vi "DtCreateAoutRawChan.vi"(2 "Range Min":dbl=-10.0, 3 "Range Max":dbl=10.0, 5 "Board Name":string, 7 "Channel":string="0", 9 "Element":u32, 11 "error in (no error)":errorcluster) -> (4 "Task out":i32, 8 "Actual Number of Channels":u32, 15 "error out":errorcluster)   [LabVIEW 2016]
doc: "Creates one or more virtual analog output channels to output raw counts. If your device supports streaming digital outputs through the analog output subsystem, this VI also creates one or more virtual channels for the digital output ports.\n\nLV-Link automatically configures the appropriate data encoding (binary or twos complement) and resolution for the subsystem, and sets the gain for all analog output channels to 1.\n\nYou can update the value of one or more virtual analog output channels using the DtOLWrite VI."
uses:
  <userlib>/LV-Link3/DtLvLink.lvlib
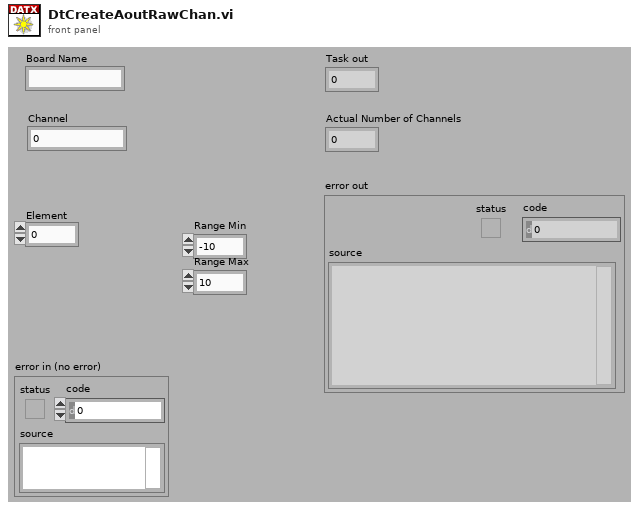
[diagram p1: front panel]
types:
  T1 = enum32{"AnalogInput", "AnalogOutput", "DigitalInput", "DigitalOutput", "Quadrature", "CounterTimer"}
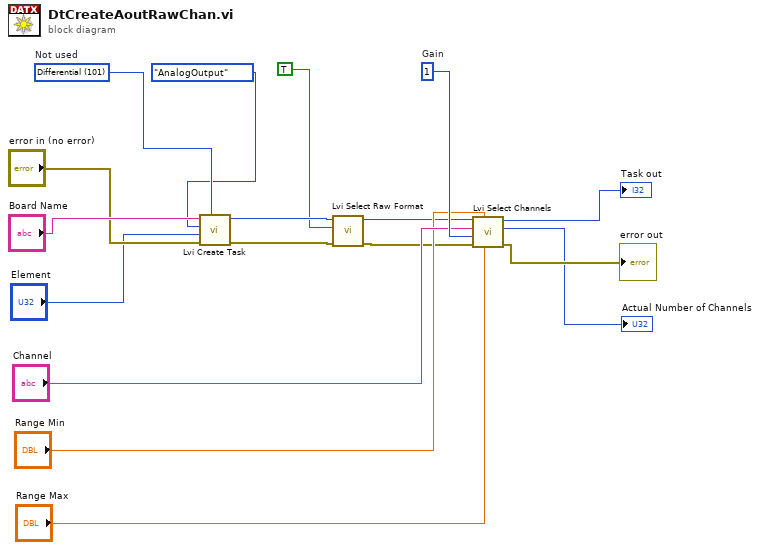
[diagram p0: block diagram]
diagram:
  w8 = 101 items=["SingleEnded"=100, "Differential"=101]  # Not used
  w17 = u32 1  # Gain
  n1 = call <userlib>:"Lvi Create Task.vi"("SEorDiff"=w8, "error in (no error)"="error in (no error)", "SubSysIndex"="Element", "ChanType"=T1."AnalogOutput", "BoardName"="Board Name") -> ("error out"=w6:errorcluster, "TaskRef"=w7:i32)  [unwired: 4 in, 1 out]
  n2 = call <userlib>:"Lvi Select Raw Format.vi"("error in (no error)"=w6, "RawFormat"=TRUE ("Boolean RawFormat"), "TaskRef"=w7) -> ("error out"=w5:errorcluster, "TaskRef out"=w1:i32)  [unwired: 6 in, 1 out]
  n3 = call <userlib>:"Lvi Select Channels.vi"("MaxRange"="Range Max", "MinRange"="Range Min", "error in (no error)"=w5, "Gain"=w17, "ChanListStr"="Channel", "TaskRef"=w1) -> ("error out"=→"error out":errorcluster, "ActualNumChannels"=→"Actual Number of Channels":u32, "TaskRef out"=→"Task out":i32)  [unwired: 2 in, 1 out]
